vi "H3 do it yourself.vi"() -> ()   [LabVIEW 2017]
uses:
  <vilib>/Analysis/NI_AALBase.lvlib
panel:
  out "Waveform Graph":i32[](graph)
  in  "total number of trails":dbl
  out "number of heads":dbl
  out "coin 4":bool
  out "coin 3":bool
  out "coin 2":bool
  out "coin 1":bool
  # "tails = unlit"
  # "heads = lit"
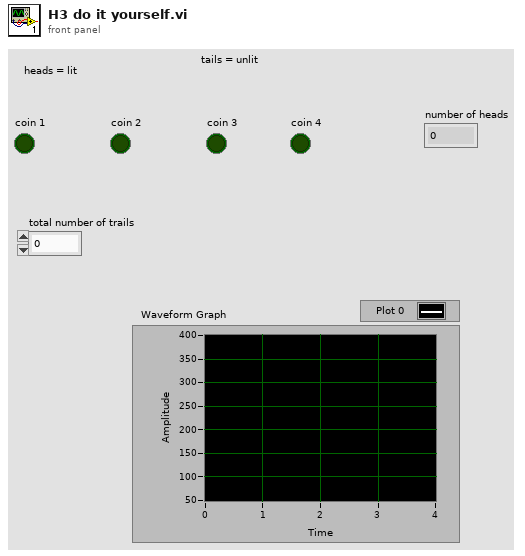
[diagram p1: front panel]
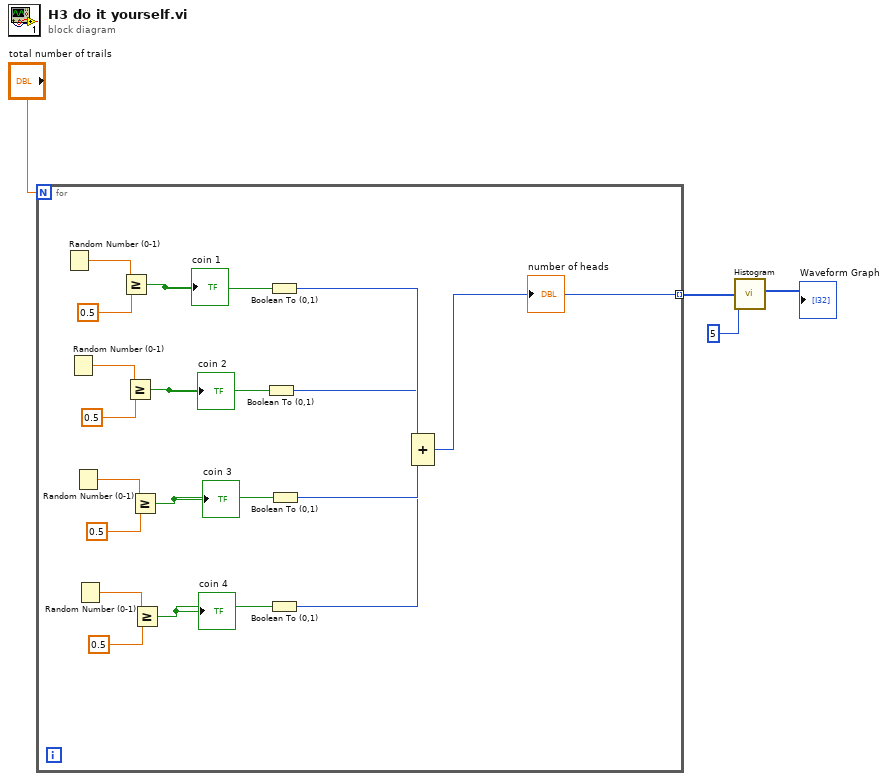
[diagram p0: block diagram]
diagram:
  n1 = for {
    N: "total number of trails" -> [_]
    tunnel: [w5] -> w2 mode=indexing
    n2 = Random Number (0-1)() -> (number: 0 to 1=w21:dbl)
    n3 = Random Number (0-1)() -> (number: 0 to 1=w18:dbl)
    n4 = Random Number (0-1)() -> (number: 0 to 1=w16:dbl)
    n5 = Random Number (0-1)() -> (number: 0 to 1=w14:dbl)
    n6 = Greater Or Equal?(x=w21, y=0.5) -> (x >= y?=w19:bool)
    "coin 1" <- w19
    n7 = Greater Or Equal?(x=w18, y=0.5) -> (x >= y?=w12:bool)
    "coin 2" <- w12
    n8 = Greater Or Equal?(x=w16, y=0.5) -> (x >= y?=w11:bool)
    "coin 3" <- w11
    n9 = Greater Or Equal?(x=w14, y=0.5) -> (x >= y?=w10:bool)
    "coin 4" <- w10
    n10 = Boolean To (0,1)(Boolean=w12) -> (0, 1=w8:i16)
    n11 = Boolean To (0,1)(Boolean=w19) -> (0, 1=w9:i16)
    n12 = Boolean To (0,1)(Boolean=w10) -> (0, 1=w6:i16)
    n13 = Boolean To (0,1)(Boolean=w11) -> (0, 1=w7:i16)
    n14 = Compound Arithmetic op=ADD(w9, w8, w7, w6) -> (w5:i16)
    "number of heads" <- w5
  }
  n15 = call <vilib>:"Histogram.vi"("intervals"=5, "X"=w2) -> ("Histogram: h(x)"=→"Waveform Graph":i32[])  [unwired: 6 in, 3 out]
